vi "Calibration Adjust Count Query.vi"(8 "error in (no error)":errorcluster, 11 "VISA resource name":refnum<visa-resource-name>="GPIB0::24::INSTR") -> (0 "error out":errorcluster, 2 "Cal Count":i32, 3 "VISA resource name out":refnum<visa-resource-name>)   [LabVIEW 2022 SP3, in "Keithley 2450.lvlib"]
doc: "This VI queries calibration adjust count."
uses:
  Keithley 2450.lvlib
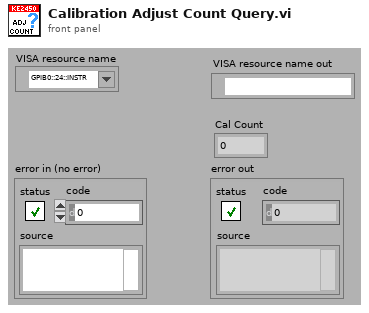
[diagram p1: front panel]
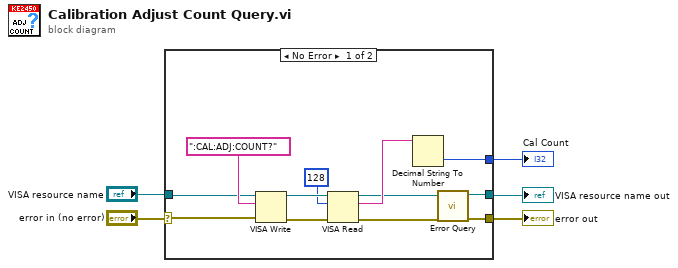
[diagram p0: block diagram]
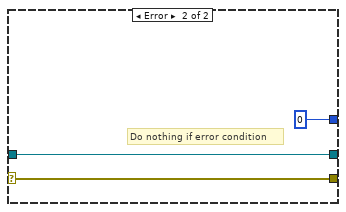
[diagram p2: hidden frame]
diagram:
  n1 = case shown="No Error" "error in (no error)" {
    selector: "error in (no error)" -> [w13 w20]
    tunnel: [w9 w20] -> w4
    tunnel: "VISA resource name" -> [w11 w19]
    tunnel: [w8 w19] -> w2
    tunnel: [w10 0] -> w1
    frame No Error {
      n2 = VISA Write(VISA resource name=w11, write buffer=":CAL:ADJ:COUNT?" ("format string"), error in (no error)=w13) -> (VISA resource name out=w16:refnum<visa-resource-name>, error out=w17:errorcluster)  [unwired: 1 out]
      n3 = VISA Read(VISA resource name=w16, byte count=u32 128, error in (no error)=w17) -> (VISA resource name out=w7:refnum<visa-resource-name>, read buffer=w14:string, error out=w6:errorcluster)  [unwired: 1 out]
      n4 = Decimal String To Number(string=w14) -> (number=w10:i32)  [unwired: 3 out]
      n5 = call "Error Query.vi"("error in (no error)"=w6, "VISA resource name"=w7) -> ("error out"=w9:errorcluster, "VISA resource name out"=w8:refnum<visa-resource-name>)  [unwired: 6 in, 2 out]
    }
    frame Error {
      # "Do nothing if error condition"
    }
  }
  "error out" <- w4
  "VISA resource name out" <- w2
  "Cal Count" <- w1
